vi "TSM DAQmx N Pins To 1 Task.vi"(0 "TSM context":T3, 5 "Pins":tag[](array[tag]), 7 "Site Numbers":i32[](array[numeric]), 11 "error in":errorcluster) -> (4 "DAQ TSM Out":T1, 15 "error out":errorcluster)   [LabVIEW 2019]
uses:
  <vilib>/NI_TestStand_SemiconductorModule/NI_TestStand_Semiconductor_Module.lvlibp/PinMap/General/SemiconductorModuleContext.ctl
  TSM DAQmx.ctl
  <vilib>/NI_TestStand_SemiconductorModule/NI_TestStand_Semiconductor_Module.lvlibp/PinMap/PinQueryContext/MultiplePinSingleSessionQueryContext/MultiplePinSingleSessionQueryContext.lvclass
  SSC DAQmx.ctl
  <vilib>/NI_TestStand_SemiconductorModule/NI_TestStand_Semiconductor_Module.lvlibp/PinMap/DAQmx/PinsToNIDAQmxTask.vi
  <vilib>/NI_TestStand_SemiconductorModule/NI_TestStand_Semiconductor_Module.lvlibp
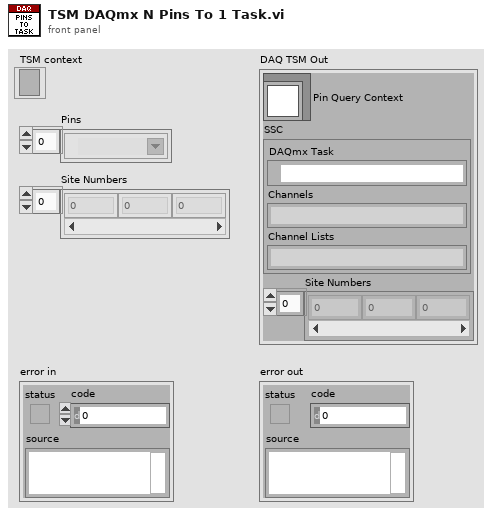
[diagram p1: front panel]
types:
  T1 = typedef "TSM DAQmx.ctl" = cluster{"Pin Query Context":refnum<class "MultiplePinSingleSessionQueryContext.lvclass">, "SSC":T2, "Site Numbers":i32[]}
  T2 = typedef "SSC DAQmx.ctl" = cluster{"DAQmx Task ":refnum<k21>, "Channels":string, "Channel Lists":string}
  T3 = typedef "NI_TestStand_Semiconductor_Module.lvlibp/SemiconductorModuleContext.ctl" = refnum<k7>
  T4 = cluster{"DAQmx Task":refnum<k21>, "Channel List":string, "spreadsheet string":string}
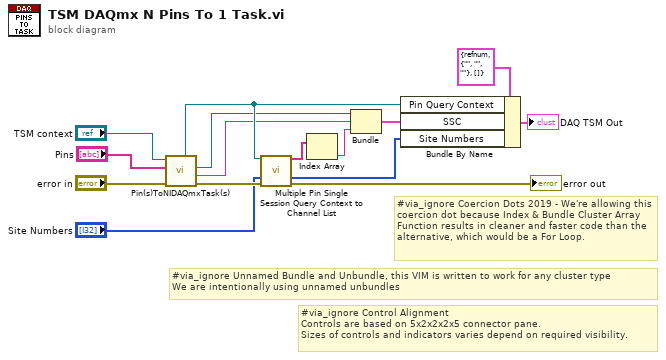
[diagram p0: block diagram]
diagram:
  # "#via_ignore Coercion Dots 2019 - We're allowing this coercion dot because Index & Bundle Cluster Array Function results in cleaner and faster code than the alternative, which would be a For Loop."
  # "#via_ignore Unnamed Bundle and Unbundle, this VIM is written to work for any cluster type\nWe are intentionally using unnamed unbundles"
  # "#via_ignore Control Alignment\nControls are based on 5x2x2x2x5 connector pane.\nSizes of controls and indicators varies depend on required visibility."
  n1 = call-poly <vilib>:"Pin(s)ToNIDAQmxTask(s).vi"("error in (no error)"="error in", "Pins"="Pins", "Semiconductor Module Context"="TSM context") -> ("error out"=w13:errorcluster, "Channel List"=w2:string, "DAQmx Task"=w3:refnum<k21>, "Pin Query Context"=w6:refnum<class "MultiplePinSingleSessionQueryContext.lvclass">)  [unwired: 4 in, 1 out]
  n2 = call "Multiple Pin Single Session Query Context to Channel List.vi"("Multiple Pin Single Session Query Context"=w6, "Site Numbers In"="Site Numbers", "error in"=w13) -> ("Per-Session Channel List"=w5:string[], "Site Numbers Out"=w8:i32[], "error out"=→"error out":errorcluster)  [unwired: 10 in]
  n3 = Index Array(array=w5) -> (element=w4:string)  [unwired: 1 in]
  n4 = Bundle("DAQmx Task"=w3, "Channel List"=w2, "spreadsheet string"=w4) -> (w1:T4)  [unwired: 1 in]
  n5 = Bundle By Name(cluster=T1 {"Pin Query Context"=refnum, "SSC"={"DAQmx Task "="", "Channels"="", "Channel Lists"=""}, "Site Numbers"=[]} ("DAQ TSM Out 2"), "Pin Query Context"=w6, "SSC"=w1, "Site Numbers"=w8) -> (→"DAQ TSM Out":T1)
